vi "Config ACTION.vi"(8 "error in (no error)":errorcluster, 11 "Measurement wMaster in":refnum<class "Measurement wMaster.lvclass">) -> (0 "error out":errorcluster, 3 "Measurement wMaster out":refnum<class "Measurement wMaster.lvclass">)   [LabVIEW 2014, in "SeqLoop.lvlib" / "STEP Classes.lvlib" / "Measurement wMaster.lvclass"]
uses:
  Measurement wMaster.lvclass
  Resources/XControls/Selectable ListBox xControl/ListBox XControl.xctl
  <vilib>/Utility/miscctls.llb/LVPointTypeDef.ctl
  Measurement wMaster.lvclass/Measurement wMaster.ctl
panel:
  in  "Deselect All":bool
  in  "Select All":bool
  in  "Cancel":bool
  in  "Save":bool
  in  "Measurement List":string[](xcontrol)
  in  "HWAsync Actions":T1={"HWAsync 1"="---", "HWAsync 2"="---", "HWAsync 3"="---", "HWAsync 4"="---", "HWAsync 5"="---", "HWAsync 6"="---", "HWAsync 7"="---", "HWAsync 8"="---", "HWAsync 9"="---", "HWAsync 10"="---"}
  # "Seleccione Mediciones a Calcular"
  # "Hardware Asíncronos"
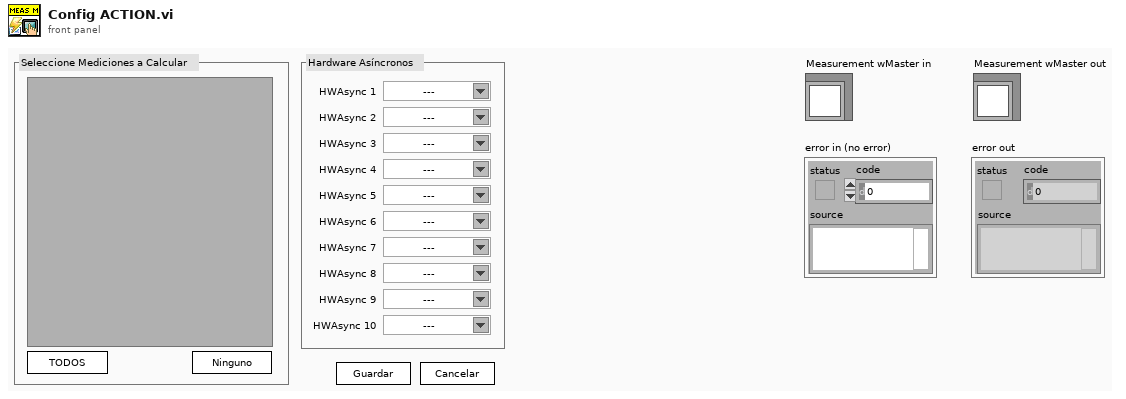
[diagram p1: front panel]
types:
  T1 = cluster{"HWAsync 1":string, "HWAsync 2":string, "HWAsync 3":string, "HWAsync 4":string, "HWAsync 5":string, "HWAsync 6":string, "HWAsync 7":string, "HWAsync 8":string, "HWAsync 9":string, "HWAsync 10":string}
  T2 = typedef "LVPointTypeDef.ctl" = cluster{"Horizontal":i16, "Vertical":i16}
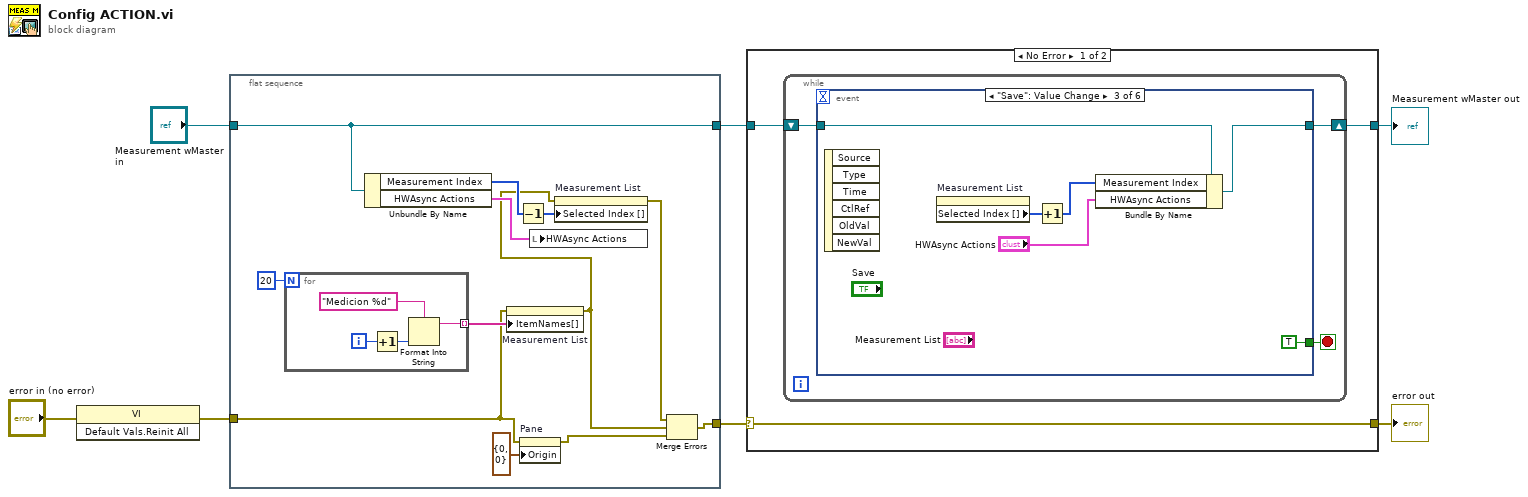
[diagram p0: block diagram]
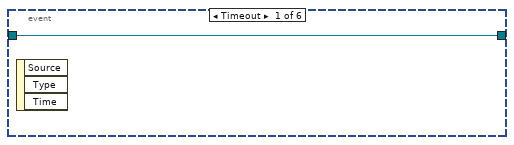
[diagram p2: hidden frame]
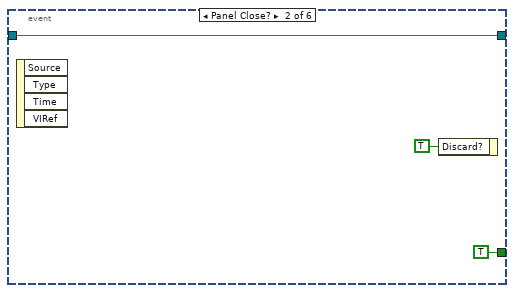
[diagram p3: hidden frame]
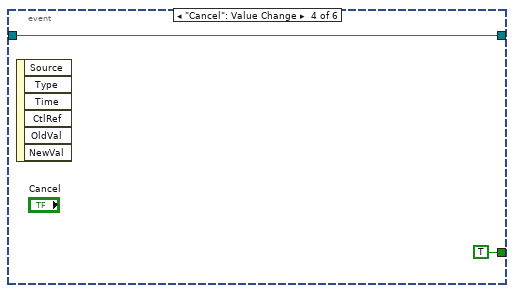
[diagram p4: hidden frame]
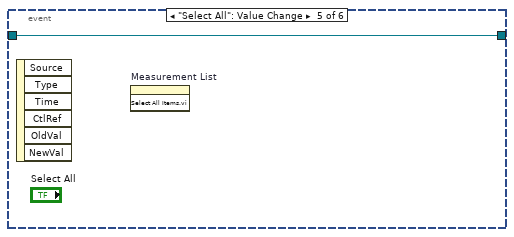
[diagram p5: hidden frame]
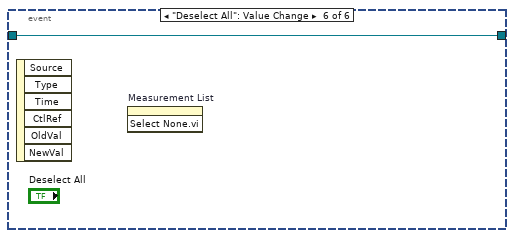
[diagram p6: hidden frame]
diagram:
  n1 = invoke class="VI" method="Default Vals.Reinit All"(error in="error in (no error)") -> (error out=w6:errorcluster)  [unwired: 2 in, 2 out]
  n2 = flat-sequence {
    tunnel: "Measurement wMaster in" -> [w13]
    tunnel: [w17] -> w7
    tunnel: w6 -> [w9]
    tunnel: [w13] -> w5
    frame #0 {
      n3 = for {
        N: 20 -> [_]
        tunnel: [w20] -> w19 mode=indexing
        i -> [w21]
        n4 = Increment(x=w21) -> (x+1=w22:i32)
        n5 = Format Into String(format string="Medicion %d", w22) -> (resulting string=w20:string)  [unwired: 2 in, 1 out]
      }
      n6 = Unbundle By Name(w13) -> ("Measurement Index"=w14:i32[], "HWAsync Actions"=w10:T1)
      n7 = property on="Measurement List" class="ListBox XControl (strict)"(error in=w9, "ItemNames[]"=w19) -> (error out=w8:errorcluster)  [unwired: 1 in, 1 out]
      n8 = Decrement(x=w14) -> (x-1=w15:i32[])
      n9 = property on="Pane" class="Pane"(error in=w9, "Origin"=T2 {"Horizontal"=0, "Vertical"=0}) -> (error out=w11:errorcluster)  [unwired: 1 in, 1 out]
      n10 = local write "HWAsync Actions"(w10) -> ()
      n11 = property on="Measurement List" class="ListBox XControl (strict)"(error in=w8, "Selected Index []"=w15) -> (error out=w16:errorcluster)  [unwired: 1 in, 1 out]
      n12 = Merge Errors(w16, w8, w11) -> (w17:errorcluster)
    }
  }
  n13 = case shown="No Error" w7 {
    selector: w7 -> [w26 w45]
    tunnel: [w26 w45] -> w1
    tunnel: [w24 w44] -> w2
    tunnel: w5 -> [w25 w44]
    frame No Error {
      n14 = while {
        shift-right: [w28] -> w24
        shift-left: w25 -> [w29]
        stop <- w27 stop-if-true
        n15 = event shown="[2] \"Save\": Value Change" {
          selector: _ -> [_ _ _ _ _ _]
          dyn-events: _ -> [_ _ _ _ _ _]
          timeout: _ -> [_ _ _ _ _ _]
          tunnel: w29 -> [w30 w33 w37 w41 w42 w43]
          tunnel: [w30 w33 w36 w41 w42 w43] -> w28
          tunnel: [_ TRUE TRUE TRUE _ _] -> w27
          event Timeout {
            n16 = event-data() -> ()  [unwired: 1 in, 3 out]
          }
          event Panel Close? {
            n17 = event-data() -> ()  [unwired: 1 in, 4 out]
            n18 = event-data("Discard?"=TRUE) -> ()  [unwired: 1 in, 1 out]
          }
          event "Save": Value Change {
            n19 = event-data() -> ()  [unwired: 1 in, 6 out]
            n20 = property on="Measurement List" class="ListBox XControl (strict)"() -> ("Selected Index []"=w35:i32[])  [unwired: 2 in, 2 out]
            n21 = Increment(x=w35) -> (x+1=w34:i32[])
            n22 = Bundle By Name(cluster=w37, "Measurement Index"=w34, "HWAsync Actions"="HWAsync Actions") -> (w36:refnum<class "Measurement wMaster.lvclass">)
          }
          event "Cancel": Value Change {
            n23 = event-data() -> ()  [unwired: 1 in, 6 out]
          }
          event "Select All": Value Change {
            n24 = event-data() -> ()  [unwired: 1 in, 6 out]
            n25 = invoke on="Measurement List" class="ListBox XControl (strict)" method="Select All Items.vi"() -> ()  [unwired: 3 in, 3 out]
          }
          event "Deselect All": Value Change {
            n26 = event-data() -> ()  [unwired: 1 in, 6 out]
            n27 = invoke on="Measurement List" class="ListBox XControl (strict)" method="Select None.vi"() -> ()  [unwired: 3 in, 3 out]
          }
        }
      }
    }
    frame Error {
    }
  }
  "error out" <- w1
  "Measurement wMaster out" <- w2
